vi "OpenDevice.vi"(11 "error in":errorcluster caption="错误输入") -> (3 "error out":errorcluster caption="错误输出")   [LabVIEW 2016]
uses:
  PLC-Lab/lib/gusb.dll
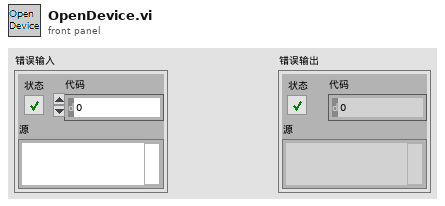
[diagram p1: front panel]
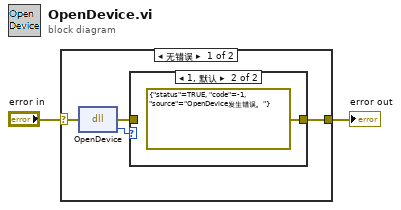
[diagram p0: block diagram]
diagram:
  n1 = case shown="无错误" "error in" {
    selector: "error in" -> [w6 w9]
    tunnel: [w3 w9] -> w1
    frame No Error {
      n2 = dll-call lib="E:/Camproject/2018/2018.1Labview/PLC-Lab/lib/gusb.dll" fn="OpenDevice"(error in=w6) -> (error out=w4:errorcluster, "Status"=w5:i32)  [unwired: 2 in, 1 out]
      n3 = case shown="1, 默认" w5 {
        tunnel: w4 -> [w7 _]
        tunnel: [w7 errorcluster {"status"=TRUE, "code"=-1, "source"="OpenDevice发生错误。"} ("错误常量")] -> w3
        frame 0 {
        }
        frame 1, Default {
        }
      }
    }
    frame Error {
    }
  }
  "error out" <- w1
